vi "S8300E_RTC_SFCS_Compare.vi"() -> ()   [LabVIEW 2011]
uses:
  Instance          11 29Saved   Mojo_RTC_SFCS_Compare .vi
  Instance           1 29Saved   Mojo_RTC_SFCS_Compare .vi
  Instance           4 29Saved   Mojo_RTC_SFCS_Compare .vi
  Instance           2 29Saved   Mojo_RTC_SFCS_Compare .vi
  data/MCSDLL.dll
panel:
  out "Tolerance sec":string
  out "UUT sec":i32
  out "UUT min":i32
  out "UUT hour":i32
  out "UUT Day":i32
  out "UUT  Month":i32
  out "UUT Year":i32
  out "UUT-DateTime":string
  out "VISA resource name out":refnum<visa-resource-name>
  out "Start Time":u32
  out "Tolerance_sec_gap":dbl
  out "TimeGap(sec)":dbl format="%#_8f"
  out "sec":i32
  out "minute":i32
  out "hour":i32
  out "day":i32
  out "month":i32
  out "year":i32
  out "SFCS_Time":string
  out "SFCS_DATE_STRING":string
  out "output param":string
  out "STAGE":string
  out "SFCS_IP":string
  in  "URL":string
  # "Error Code:RTC\nError Code:UART"
  # "網路時間與S8300E 時間比較\nNetwork Time compare to S8300E RTC Time"
  # "2014-12-15"
  # "COM9, Baud 115200"
  # "SFCS Time:"
  # "UUT-Date-Time:"
  # "Formula :TimeGap=SFCS Time-UUT Time"
  # "<"
  # "Pass Criteria"
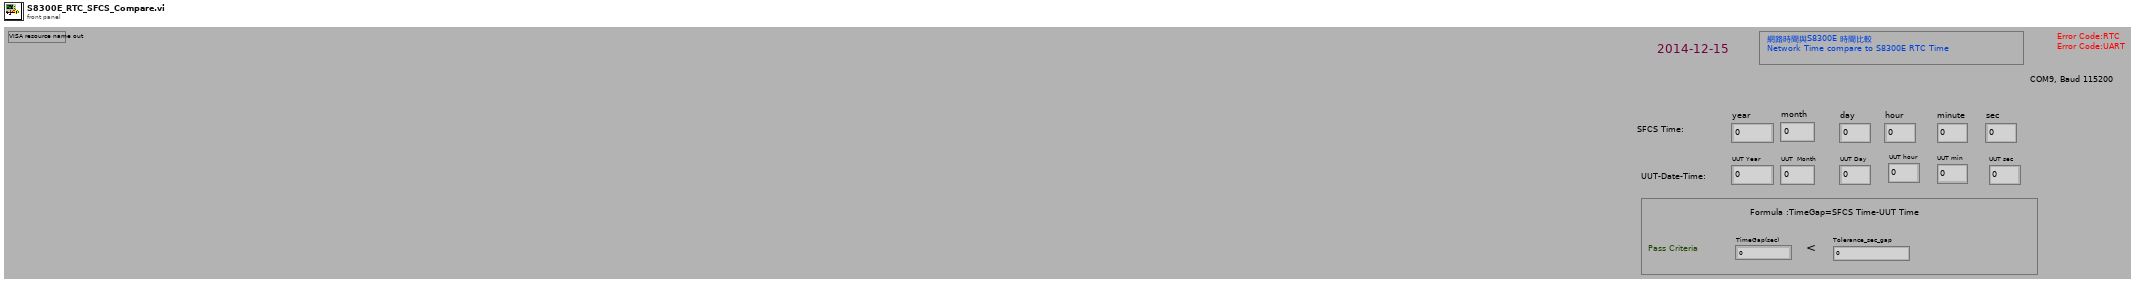
[diagram p1: front panel]
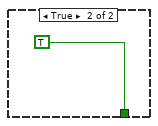
[diagram p5: hidden frame]
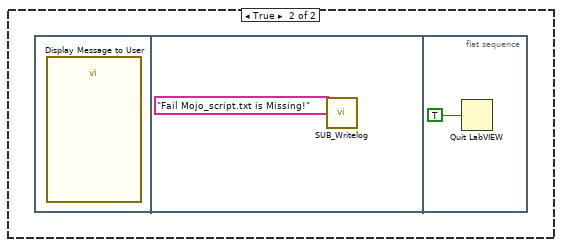
[diagram p7: hidden frame]
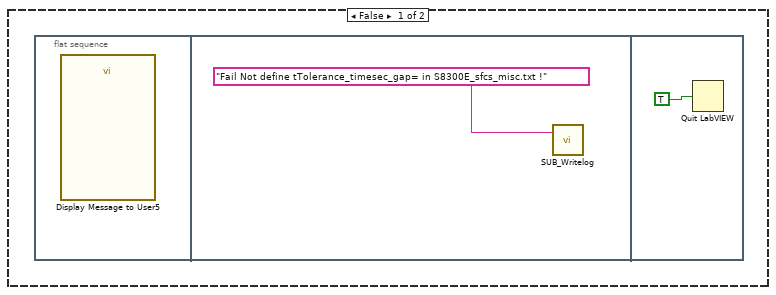
[diagram p8: hidden frame]
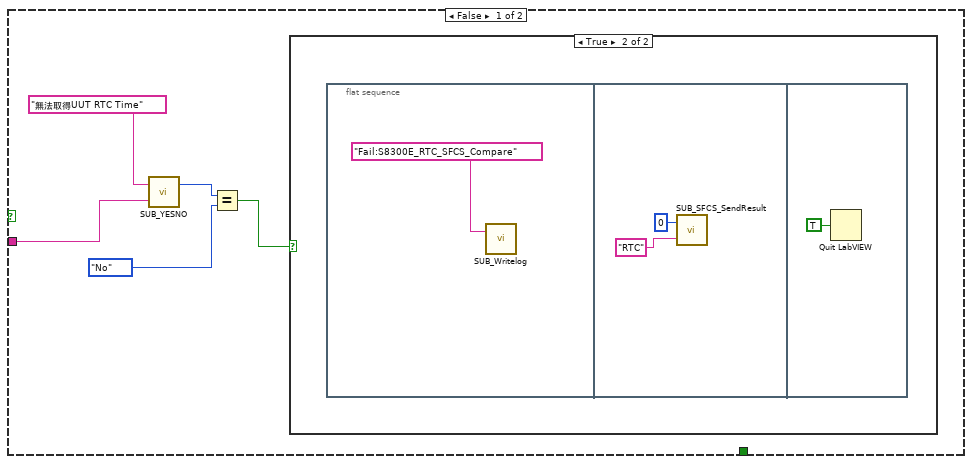
[diagram p10: hidden frame]
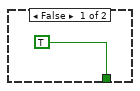
[diagram p12: hidden frame]
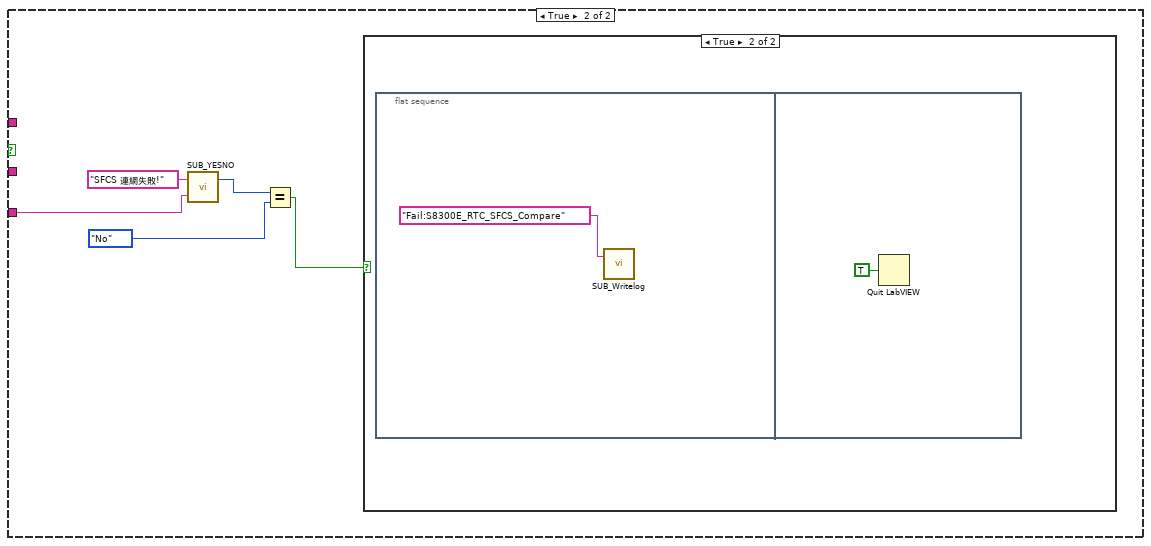
[diagram p14: hidden frame]
diagram:
  n1 = flat-sequence {
    tunnel: [w34] -> w2
    tunnel: w2 -> [w57]
    tunnel: [w57] -> w1
    tunnel: w1 -> [w65]
    frame #0 {
      n2 = Tick Count (ms)() -> (millisecond timer value=→"Start Time":u32)
    }
    frame #1 {
      n3 = call "SUB_COM1_CLOSE.vi"("VISA resource name"=refnum<visa-resource-name> "COM9") -> ()  [unwired: 3 in]
    }
    frame #2 {
      n4 = case shown="True" TRUE {
        frame False {
        }
        frame True {
          n5 = call "SUB_COM9_INIT.vi"("baud rate"=u32 115200) -> ("VISA resource name out"=w9:refnum<visa-resource-name>)  [unwired: 1 in, 1 out]
          "VISA resource name out" <- w9
          n6 = call "SUB_COM1Wrt.vi"("VISA resource name"=w9, "write buffer"="\r") -> ("duplicate VISA resource name"=w6:refnum<visa-resource-name>)  [unwired: 1 in, 1 out]
          n7 = call "SUB_ContinueCom1Read.vi"("Numeric"=1200, "duplicate VISA resource name 2"=w6) -> ()  [unwired: 1 in, 3 out]
        }
      }
    }
    frame #3 {
      n8 = case shown="True" TRUE {
        frame False {
        }
        frame True {
          n9 = while {
            stop <- w19 stop-if-true
            n10 = local read "VISA resource name out"() -> (w18:refnum<visa-resource-name>)
            n11 = Tick Count (ms)() -> (millisecond timer value=w13:u32)
            n12 = call "SUB_COM1Wrt.vi"("VISA resource name"=w18, "write buffer"="\r") -> ("duplicate VISA resource name"=w14:refnum<visa-resource-name>)  [unwired: 1 in, 1 out]
            n13 = call "SUB_READ_COM1_FindString_timeout.vi"("Find this String"="S8300E", "Timeout Seccond"=2.0, "Begin time"=w13, "duplicate VISA resource name 2"=w14) -> ("Output String"=w16:string, "Found String"=w15:bool)  [unwired: 1 in, 1 out]
            n14 = case shown="False" w15 {
              tunnel: w16 -> [w25 _]
              tunnel: [w21 TRUE] -> w19
              frame False {
                n15 = call "SUB_YESNO.vi"("Debug View"=w25, "Status"="UART無正確反應!需有S8300E字串") -> ("yes/no"=w24:enum32{"No Selection", "Yes", "No", "None"})  [unwired: 1 in]
                n16 = Equal?(x=w24, y=enum32{"No Selection", "Yes", "No", "None"}."No") -> (x = y?=w22:bool)
                n17 = case shown="True" w22 {
                  tunnel: [_ w27] -> w21
                  frame False {
                  }
                  frame True {
                    n18 = flat-sequence {
                      tunnel: [w31] -> w27
                      frame #0 {
                        n19 = call "SUB_Writelog.vi"("Pass/Fail"="Fail:S8300E_RTC_SFCS_Compare") -> ()  [unwired: 2 in]
                      }
                      frame #1 {
                        n20 = call "SUB_SFCS_SendResult.vi"("ErrorCode"="UART", "PASS_Fail (1/0)"=i8 0) -> ()  [unwired: 1 out]
                      }
                      frame #2 {
                        w31 = TRUE ("quit? (T)")
                        n21 = Quit LabVIEW(quit? (T)=w31) -> ()
                      }
                    }
                  }
                }
              }
              frame True {
              }
            }
          }
        }
      }
    }
    frame #4 {
      n22 = call "SUB_Read_specifFile.vi"("name or relative path"="S8300E_sfcs_misc.txt" ("Script FileName")) -> ("error out"=w37:errorcluster, "text"=w34:string)  [unwired: 1 in]
      n23 = Unbundle By Name(w37) -> ("code"=w36:i32)
      n24 = Not Equal To 0?(x=w36) -> (x != 0?=w35:bool)
      n25 = case shown="False" w35 {
        tunnel: w34 -> [w38 _]
        frame False {
          n26 = flat-sequence {
            tunnel: w38 -> [w44]
            frame #0 {
              n27 = To Upper Case(1:"SFCS_IP=" ("string")) -> (0:w48:string)
              n28 = To Upper Case(1:w44) -> (0:w49:string)
              n29 = call <vilib>:"Trim Whitespace.vi"("string"=w48) -> ("trimmed string"=w46:string)  [unwired: 1 in]
              n30 = call <vilib>:"Trim Whitespace.vi"("string"=w49) -> ("trimmed string"=w45:string)  [unwired: 1 in]
              n31 = Match Pattern(string=w45, regular expression=w46) -> (after substring=w43:string)  [unwired: 1 in, 3 out]
              n32 = Match Pattern(string=w43, regular expression=";") -> (before substring=w41:string)  [unwired: 1 in, 3 out]
              "SFCS_IP" <- w41
              n33 = Equal?(x=w41, y="") -> (x = y?=w39:bool)
              n34 = case shown="True" w39 {
                frame False {
                }
                frame True {
                  n35 = flat-sequence {
                    frame #0 {
                      n36 = call "Display Message to User2"() -> ()  [unwired: 10 in, 2 out]
                    }
                    frame #1 {
                      n37 = call "SUB_Writelog.vi"("Pass/Fail"="Fail Not Found SFCS_IP=\"xx.xx.xx.xx\" in S8300E_sfcs_misc.txt !") -> ()  [unwired: 2 in]
                    }
                    frame #2 {
                      n38 = Quit LabVIEW(quit? (T)=TRUE) -> ()
                    }
                  }
                }
              }
            }
          }
        }
        frame True {
          n39 = flat-sequence {
            frame #0 {
              n40 = call "Display Message to User"() -> ()  [unwired: 10 in, 2 out]
            }
            frame #1 {
              n41 = call "SUB_Writelog.vi"("Pass/Fail"="Fail Mojo_script.txt is Missing!") -> ()  [unwired: 2 in]
            }
            frame #2 {
              n42 = Quit LabVIEW(quit? (T)=TRUE) -> ()
            }
          }
        }
      }
    }
    frame #5 {
      n43 = call "SUB_FindSpecificString.vi"("Find this String"="Tolerance_timesec_gap=", "String data"=w57) -> ("before \"; \" string"=w54:string, "Found"=w55:bool)  [unwired: 2 in]
      n44 = case shown="True" w55 {
        tunnel: w54 -> [_ w61]
        frame False {
          n45 = flat-sequence {
            frame #0 {
              n46 = call "Display Message to User5"() -> ()  [unwired: 10 in, 2 out]
            }
            frame #1 {
              n47 = call "SUB_Writelog.vi"("Pass/Fail"="Fail Not define tTolerance_timesec_gap= in S8300E_sfcs_misc.txt !") -> ()  [unwired: 2 in]
            }
            frame #2 {
              n48 = Quit LabVIEW(quit? (T)=TRUE) -> ()
            }
          }
        }
        frame True {
          n49 = Fract/Exp String To Number(string=w61) -> (number=→"Tolerance_sec_gap":dbl)  [unwired: 3 in, 1 out]
          "Tolerance sec" <- w61
        }
      }
    }
    frame #6 {
      n50 = To Upper Case(1:"SFCS_STAGE=" ("string")) -> (0:w71:string)
      n51 = To Upper Case(1:w65) -> (0:w72:string)
      n52 = call <vilib>:"Trim Whitespace.vi"("string"=w71) -> ("trimmed string"=w70:string)  [unwired: 1 in]
      n53 = call <vilib>:"Trim Whitespace.vi"("string"=w72) -> ("trimmed string"=w69:string)  [unwired: 1 in]
      n54 = Match Pattern(string=w69, regular expression=w70) -> (after substring=w68:string)  [unwired: 1 in, 3 out]
      n55 = Match Pattern(string=w68, regular expression=";") -> (before substring=w64:string)  [unwired: 1 in, 3 out]
      "STAGE" <- w64
      n56 = Not Equal?(x=w64, y="") -> (x != y?=w62:bool)
      n57 = case shown="False" w62 {
        frame False {
          n58 = flat-sequence {
            frame #0 {
              n59 = call "Display Message to User4"() -> ()  [unwired: 10 in, 2 out]
            }
            frame #1 {
              n60 = call "SUB_Writelog.vi"("Pass/Fail"="Fail :Stage  not define in script file!") -> ()  [unwired: 2 in]
            }
            frame #2 {
              n61 = Quit LabVIEW(quit? (T)=TRUE) -> ()
            }
          }
        }
        frame True {
        }
      }
    }
    frame #7 {
      n62 = while {
        stop <- w80 stop-if-true
        n63 = Concatenate Strings("./rtc.sh -r" ("string"), "\r") -> (w86:string)
        n64 = Tick Count (ms)() -> (millisecond timer value=w76:u32)
        n65 = local read "VISA resource name out"() -> (w84:refnum<visa-resource-name>)
        n66 = call "SUB_COM1Wrt.vi"("VISA resource name"=w84, "write buffer"=w86) -> ("duplicate VISA resource name"=w77:refnum<visa-resource-name>)  [unwired: 1 in, 1 out]
        n67 = call "SUB_READ_COM1_FindString_timeout.vi"("Find this String"="PASSED=", "Timeout Seccond"=3.0, "Begin time"=w76, "duplicate VISA resource name 2"=w77) -> ("Output String"=w79:string)  [unwired: 1 in, 2 out]
        n68 = call "SUB_FindSpecificString.vi"("Find this String"="PASSED=", "String data"=w79) -> ("before \"; \" string"=→"UUT-DateTime":string, "Found"=w81:bool)  [unwired: 2 in]
        n69 = case shown="True" w81 {
          tunnel: w79 -> [w91 _]
          tunnel: [_ TRUE] -> w80
          frame False {
            n70 = call "SUB_YESNO.vi"("Debug View"=w91, "Status"="無法取得UUT RTC Time") -> ("yes/no"=w90:enum32{"No Selection", "Yes", "No", "None"})  [unwired: 1 in]
            n71 = Equal?(x=w90, y=enum32{"No Selection", "Yes", "No", "None"}."No") -> (x = y?=w88:bool)
            n72 = case shown="True" w88 {
              frame False {
              }
              frame True {
                n73 = flat-sequence {
                  frame #0 {
                    n74 = call "SUB_Writelog.vi"("Pass/Fail"="Fail:S8300E_RTC_SFCS_Compare") -> ()  [unwired: 2 in]
                  }
                  frame #1 {
                    n75 = call "SUB_SFCS_SendResult.vi"("ErrorCode"="RTC", "PASS_Fail (1/0)"=i8 0) -> ()  [unwired: 1 out]
                  }
                  frame #2 {
                    n76 = Quit LabVIEW(quit? (T)=TRUE) -> ()
                  }
                }
              }
            }
          }
          frame True {
          }
        }
      }
    }
    frame #8 {
      n77 = local read "UUT-DateTime"() -> (w104:string)
      n78 = call "SUB_UUT_DatTime_Display.vi"("UUT_DateTime_input"=w104) -> ("UUT sec"=→"UUT sec":i32, "UUT min"=→"UUT min":i32, "UUT hour"=→"UUT hour":i32, "UUT Day"=→"UUT Day":i32, "UUT  Month"=→"UUT  Month":i32, "UUT Year"=→"UUT Year":i32)
    }
    frame #9 {
      n79 = local read "SFCS_IP"() -> (w105:string)
      n80 = local write "URL"(w105) -> ()
    }
    frame #10 {
      n81 = while {
        stop <- w106 stop-if-true
        n82 = local read "STAGE"() -> (w119:string)
        n83 = dll-call lib="D:/S8300E_Project/data/MCSDLL.dll" fn="SFCS_GetCurrentDBSysdate"("URL"="URL", "Stage"=w119, "TimeFormat"="YYYY/MM/DD HH24:MI:SS") -> (w107:string)  [unwired: 6 in, 2 out]
        "output param" <- w107
        n84 = To Upper Case(1:"FAIL" ("string")) -> (0:w114:string)
        n85 = To Upper Case(1:"NG" ("string")) -> (0:w125:string)
        n86 = To Upper Case(1:w107) -> (0:w126:string)
        n87 = call <vilib>:"Trim Whitespace.vi"("string"=w114) -> ("trimmed string"=w111:string)  [unwired: 1 in]
        n88 = call <vilib>:"Trim Whitespace.vi"("string"=w125) -> ("trimmed string"=w122:string)  [unwired: 1 in]
        n89 = call <vilib>:"Trim Whitespace.vi"("string"=w126) -> ("trimmed string"=w115:string)  [unwired: 1 in]
        n90 = Match Pattern(string=w107, regular expression=" ") -> (before substring=w117:string, after substring=w116:string)  [unwired: 1 in, 2 out]
        n91 = Match Pattern(string=w115, regular expression=w122) -> (match substring=w123:string)  [unwired: 1 in, 3 out]
        n92 = Match Pattern(string=w115, regular expression=w111) -> (match substring=w112:string)  [unwired: 1 in, 3 out]
        n93 = Equal?(x=w112, y=w111) -> (x = y?=w109:bool)
        n94 = Equal?(x=w123, y=w122) -> (x = y?=w110:bool)
        n95 = Or(x=w110, y=w109) -> (x .or. y?=w108:bool)
        n96 = case shown="False" w108 {
          tunnel: w117 -> [w139 _]
          tunnel: w116 -> [w138 _]
          tunnel: w107 -> [_ w210]
          tunnel: [w133 _] -> w106
          frame False {
            n97 = flat-sequence {
              tunnel: w139 -> [w142]
              tunnel: w138 -> [w140]
              tunnel: [w146] -> w131
              tunnel: [w145] -> w129
              tunnel: [w144] -> w127
              tunnel: [w164] -> w137
              tunnel: [w163] -> w136
              tunnel: [w162] -> w135
              tunnel: [w161] -> w132
              tunnel: w131 -> [w161]
              tunnel: [w160] -> w130
              tunnel: w129 -> [w160]
              tunnel: [w159] -> w128
              tunnel: w127 -> [w159]
              tunnel: w137 -> [w179]
              tunnel: w136 -> [w178]
              tunnel: w135 -> [w177]
              tunnel: [w184] -> w134
              tunnel: w132 -> [w182]
              tunnel: w130 -> [w181]
              tunnel: w128 -> [w180]
              tunnel: w134 -> [w188]
              tunnel: [w185] -> w133
              frame #0 {
                n98 = call <vilib>:"Trim Whitespace.vi"("string"=w142) -> ("trimmed string"=→"SFCS_DATE_STRING":string)  [unwired: 1 in]
                n99 = call <vilib>:"Trim Whitespace.vi"("string"=w140) -> ("trimmed string"=→"SFCS_Time":string)  [unwired: 1 in]
              }
              frame #1 {
                w153 = "/" ("regular expression")
                n100 = local read "SFCS_DATE_STRING"() -> (w158:string)
                n101 = Match Pattern(string=w158, regular expression=w153) -> (before substring=w157:string, after substring=w154:string)  [unwired: 1 in, 2 out]
                n102 = Match Pattern(string=w154, regular expression=w153) -> (before substring=w150:string, after substring=w148:string)  [unwired: 1 in, 2 out]
                n103 = call <vilib>:"Trim Whitespace.vi"("string"=w157) -> ("trimmed string"=w156:string)  [unwired: 1 in]
                n104 = To Upper Case(1:w156) -> (0:w155:string)
                n105 = call <vilib>:"Trim Whitespace.vi"("string"=w148) -> ("trimmed string"=w149:string)  [unwired: 1 in]
                n106 = call <vilib>:"Trim Whitespace.vi"("string"=w150) -> ("trimmed string"=w152:string)  [unwired: 1 in]
                n107 = To Upper Case(1:w149) -> (0:w147:string)
                n108 = To Upper Case(1:w152) -> (0:w151:string)
                n109 = Decimal String To Number(string=w155) -> (number=w146:i32)  [unwired: 2 in, 1 out]
                "year" <- w146
                n110 = Decimal String To Number(string=w147) -> (number=w144:i32)  [unwired: 2 in, 1 out]
                "day" <- w144
                n111 = Decimal String To Number(string=w151) -> (number=w145:i32)  [unwired: 2 in, 1 out]
                "month" <- w145
              }
              frame #2 {
                w172 = ":" ("regular expression")
                n112 = local read "SFCS_Time"() -> (w165:string)
                n113 = Match Pattern(string=w165, regular expression=w172) -> (before substring=w176:string, after substring=w173:string)  [unwired: 1 in, 2 out]
                n114 = Match Pattern(string=w173, regular expression=w172) -> (before substring=w169:string, after substring=w167:string)  [unwired: 1 in, 2 out]
                n115 = call <vilib>:"Trim Whitespace.vi"("string"=w176) -> ("trimmed string"=w175:string)  [unwired: 1 in]
                n116 = To Upper Case(1:w175) -> (0:w174:string)
                n117 = call <vilib>:"Trim Whitespace.vi"("string"=w167) -> ("trimmed string"=w168:string)  [unwired: 1 in]
                n118 = call <vilib>:"Trim Whitespace.vi"("string"=w169) -> ("trimmed string"=w171:string)  [unwired: 1 in]
                n119 = To Upper Case(1:w168) -> (0:w166:string)
                n120 = To Upper Case(1:w171) -> (0:w170:string)
                n121 = Decimal String To Number(string=w174) -> (number=w162:i32)  [unwired: 2 in, 1 out]
                "hour" <- w162
                n122 = Decimal String To Number(string=w166) -> (number=w164:i32)  [unwired: 2 in, 1 out]
                "sec" <- w164
                n123 = Decimal String To Number(string=w170) -> (number=w163:i32)  [unwired: 2 in, 1 out]
                "minute" <- w163
              }
              frame #3 {
                n124 = local read "UUT-DateTime"() -> (w183:string)
                n125 = call "SUB_TimeGAP_SFCS_RTC.vi"("SFCS year"=w182, "UUT_DateTime_input"=w183, "SFCS month"=w181, "SFCS day"=w180, "SFCS hour"=w177, "SFCS minute"=w178, "SFCS second"=w179) -> ("TimeGap(sec)"=w184:dbl)
                "TimeGap(sec)" <- w184
              }
              frame #4 {
                n126 = local read "Tolerance_sec_gap"() -> (w187:dbl)
                n127 = Greater?(x=w188, y=w187) -> (0:w186:bool)
                n128 = case shown="True" w186 {
                  tunnel: [TRUE _] -> w185
                  frame False {
                  }
                  frame True {
                    n129 = local read "TimeGap(sec)"() -> (w199:dbl)
                    n130 = local read "Tolerance sec"() -> (w194:string)
                    n131 = Number To Fractional String(number=w199) -> (F-format string=w197:string)  [unwired: 3 in]
                    n132 = Concatenate Strings("TimeGap 需小於Tolerance Gap", "\n") -> (w200:string)
                    n133 = Concatenate Strings("目前TimeGap=" ("string"), w197, "\n", "目前ToleranceGap=" ("string"), w194) -> (w193:string)
                    n134 = call "SUB_YESNO.vi"("Debug View"=w193, "Status"=w200) -> ("yes/no"=w192:enum32{"No Selection", "Yes", "No", "None"})  [unwired: 1 in]
                    n135 = Equal?(x=w192, y=enum32{"No Selection", "Yes", "No", "None"}."No") -> (x = y?=w190:bool)
                    n136 = case shown="True" w190 {
                      frame False {
                      }
                      frame True {
                        n137 = flat-sequence {
                          frame #0 {
                            n138 = call "SUB_Writelog.vi"("Pass/Fail"="Fail:S8300E_RTC_SFCS_Compare") -> ()  [unwired: 2 in]
                          }
                          frame #1 {
                            n139 = call "SUB_SFCS_SendResult.vi"("ErrorCode"="RTC", "PASS_Fail (1/0)"=i8 0) -> ()  [unwired: 1 out]
                          }
                          frame #2 {
                            n140 = Quit LabVIEW(quit? (T)=TRUE) -> ()
                          }
                        }
                      }
                    }
                  }
                }
              }
            }
          }
          frame True {
            n141 = call "SUB_YESNO.vi"("Debug View"=w210, "Status"="SFCS 連網失敗!") -> ("yes/no"=w209:enum32{"No Selection", "Yes", "No", "None"})  [unwired: 1 in]
            n142 = Equal?(x=w209, y=enum32{"No Selection", "Yes", "No", "None"}."No") -> (x = y?=w207:bool)
            n143 = case shown="True" w207 {
              frame False {
              }
              frame True {
                n144 = flat-sequence {
                  frame #0 {
                    n145 = call "SUB_Writelog.vi"("Pass/Fail"="Fail:S8300E_RTC_SFCS_Compare") -> ()  [unwired: 2 in]
                  }
                  frame #1 {
                    n146 = Quit LabVIEW(quit? (T)=TRUE) -> ()
                  }
                }
              }
            }
          }
        }
      }
    }
    frame #11 {
      n147 = call "SUB_COM1_CLOSE.vi"("VISA resource name"=refnum<visa-resource-name> "COM9") -> ()  [unwired: 3 in]
    }
    frame #12 {
      w216 = "\r"
      n148 = local read "TimeGap(sec)"() -> (w218:dbl)
      n149 = local read "UUT-DateTime"() -> (w220:string)
      n150 = Tick Count (ms)() -> (millisecond timer value=w226:u32)
      n151 = local read "Start Time"() -> (w225:u32)
      n152 = local read "output param"() -> (w222:string)
      n153 = call "SUB_CAL_TESTTIME.vi"("Test Item name"="S8300E_RTC_SFCS_Compare", "Stop tick time"=w226, "Start tick time"=w225) -> ("Test Time output"=w215:string)  [unwired: 2 in]
      n154 = Number To Fractional String(number=w218) -> (F-format string=w217:string)  [unwired: 3 in]
      n155 = Concatenate Strings("Pass :S8300E_RTC_SFCS_Compare" ("Pass/Fail"), w216, "Message From SFCS:", w222, w216, "Message From UUT:", w220, w216, "TimeGap=", w217, w216, w215) -> (w228:string)
      n156 = call "SUB_Writelog.vi"("Pass/Fail"=w228) -> ()  [unwired: 2 in]
    }
    frame #13 {
      n157 = Request Deallocation(TRUE ("flag")) -> ()
    }
    frame #14 {
      n158 = Quit LabVIEW(quit? (T)=TRUE) -> ()
    }
  }
